vi "删除MN号.vi"(8 "error in (no error)":errorcluster caption="错误输入（无错误）", 11 "簇":cluster{"MN":string, "PW":string}={"MN"="平台数据发送系统", "PW"="平台数据发送系统"}) -> (0 "error out":errorcluster caption="错误输出", 3 "删除标记":bool)   [LabVIEW 2016, in "数据传输系统-05.lvlib"]
uses:
  <vilib>/registry/registry.llb/Registry RtKey.ctl
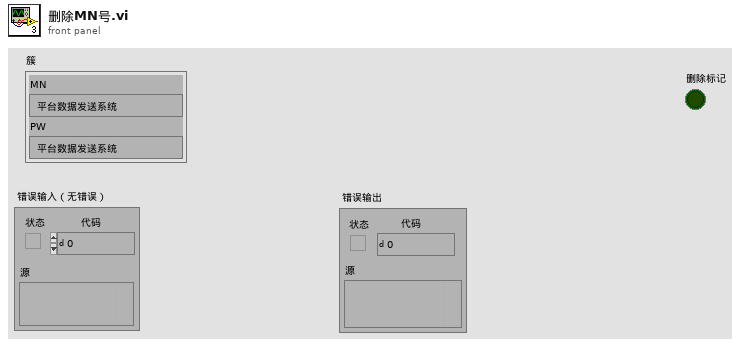
[diagram p1: front panel]
types:
  T1 = typedef "Registry RtKey.ctl" = enum32{"HKEY_CLASSES_ROOT", "HKEY_CURRENT_USER", "HKEY_LOCAL_MACHINE", "HKEY_USERS", "HKEY_PERFORMANCE_DATA", "HKEY_CURRENT_CONFIG", "HKEY_DYN_DATA"}
  T2 = typedef "Registry refnum.ctl" = refnum<k1>
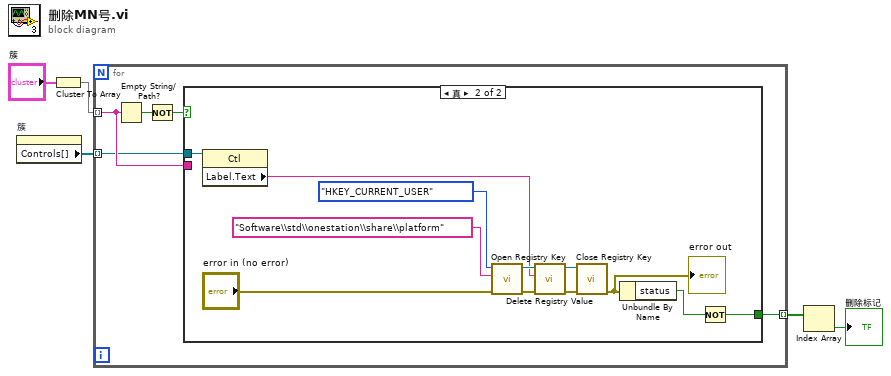
[diagram p0: block diagram]
diagram:
  n1 = property on="簇" class="Clust (严格)"() -> ("Controls[]"=w3:refnum<vi>[])  [unwired: 2 in, 2 out]
  n2 = Cluster To Array(cluster="簇") -> (array=w4:string[])
  n3 = for {
    tunnel: [w10] -> w2 mode=indexing
    tunnel: w4 -> [w7] mode=indexing
    tunnel: w3 -> [w6] mode=indexing
    n4 = Empty String/Path?(string/path=w7) -> (empty?=w9:bool)
    n5 = Not(x=w9) -> (.not. x?=w8:bool)
    n6 = case shown="真" w8 {
      tunnel: w7 -> [_ _]
      tunnel: [_ w13] -> w10
      tunnel: w6 -> [_ w12]
      frame False {
      }
      frame True {
        n7 = property class="Ctl"(reference=w12) -> ("Label.Text"=w11:string)  [unwired: 1 in, 2 out]
        n8 = call <vilib>:"Open Registry Key.vi"("error in (no error)"="error in (no error)", "subkey"="Software\\std\\onestation\\share\\platform", "root key (HKEY_LOCAL_MACHINE)"=Registry_RtKey."HKEY_CURRENT_USER") -> ("error out"=w18:errorcluster, "refnum out"=w20:T2)  [unwired: 7 in]
        n9 = call <vilib>:"Delete Registry Value.vi"("error in (no error)"=w18, "value"=w11, "refnum"=w20) -> ("error out"=w17:errorcluster, "refnum out"=w19:T2)  [unwired: 7 in]
        n10 = call <vilib>:"Close Registry Key.vi"("error in (no error)"=w17, "refnum"=w19) -> ("error out"=w15:errorcluster)  [unwired: 5 in]
        "error out" <- w15
        n11 = Unbundle By Name(w15) -> ("status"=w14:bool)
        n12 = Not(x=w14) -> (.not. x?=w13:bool)
      }
    }
  }
  n13 = Index Array(array=w2) -> (element=→"删除标记":bool)  [unwired: 1 in]
